vi "MFC WR 1 test.vi"() -> ()   [LabVIEW 2011]
uses:
  <vilib>/rvi/eio/common/nirviEmuTemplateMethod_errors.vi
  <vilib>/eio/EIOMethodNode/EIOMethodNode.xnode
panel:
  out "Time":u32
  in  "Read?":bool
  out "Array":u8[](array[numeric])
  in  "array":u8[](array[numeric])=[65, 48, 48, 48, 48, 48, 13]
  out "Timed Out":bool
  # "32000"
  # "64000"
  # "66.....73"
  # "65\n48\n48\n48\n48\n48\n13"
  # "65\n54\n52\n52\n48\n48\n13"
  # "65\n51  \n50\n48\n48\n48\n13"
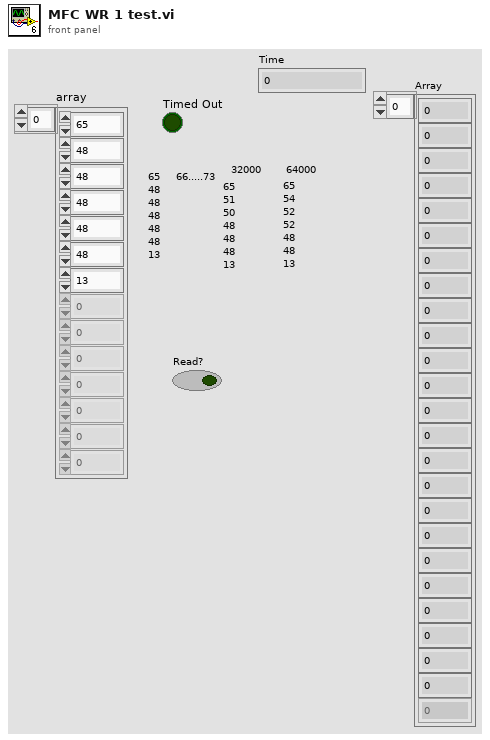
[diagram p1: front panel]
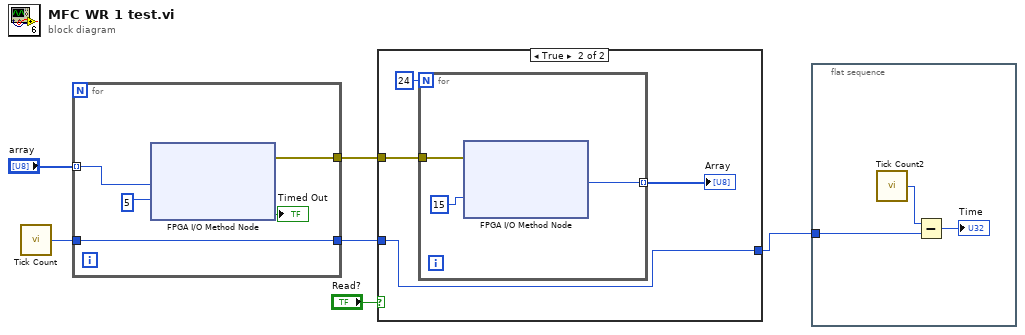
[diagram p0: block diagram]
diagram:
  n1 = call "Tick Count"() -> ("Tick Count(Ticks)"=w2:u32)
  n2 = for {
    tunnel: "array" -> [w10] mode=indexing
    tunnel: [w8] -> w5
    tunnel: [w7] -> w3
    tunnel: w2 -> [w7]
    n3 = xnode "FPGA I/O Method Node"("Data"=w10, "Timeout (ms)"=5) -> ("error out"=w8:errorcluster, "Timed Out"=→"Timed Out":bool)  [unwired: 2 in, 1 out]
  }
  n4 = case shown="True" "Read?" {
    tunnel: w5 -> [_ w16]
    tunnel: [w12 w13] -> w1
    tunnel: w3 -> [w12 w13]
    frame False {
    }
    frame True {
      n5 = for {
        N: 24 -> [_]
        tunnel: w16 -> [w19]
        tunnel: [w18] -> w15 mode=indexing
        n6 = xnode "FPGA I/O Method Node"("error in"=w19, "Timeout (ms)"=15) -> ("Data"=w18:u8)  [unwired: 1 in, 3 out]
      }
      "Array" <- w15
    }
  }
  n7 = flat-sequence {
    tunnel: w1 -> [w22]
    frame #0 {
      n8 = call "Tick Count2"() -> ("Tick Count(Ticks)"=w21:u32)
      n9 = Subtract(x=w21, y=w22) -> (x-y=→"Time":u32)
    }
  }
